vi "Read String IN.vi"(8 "error in (no error)":errorcluster, 11 "XuLyStringUART in":refnum<class "XuLyStringUART.lvclass">) -> (0 "error out":errorcluster, 2 "String IN":string, 3 "XuLyStringUART out":refnum<class "XuLyStringUART.lvclass">)   [LabVIEW 2017, in "LibraryGcode.lvlib" / "XuLyStringUART.lvclass"]
uses:
  XuLyStringUART.lvclass
  XuLyStringUART.lvclass/XuLyStringUART.ctl
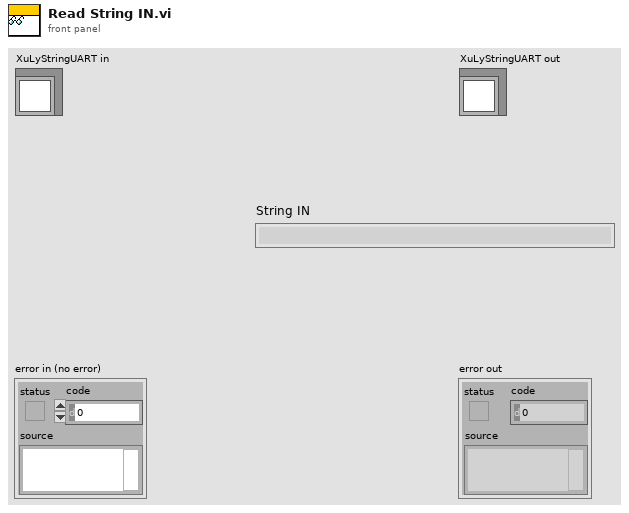
[diagram p1: front panel]
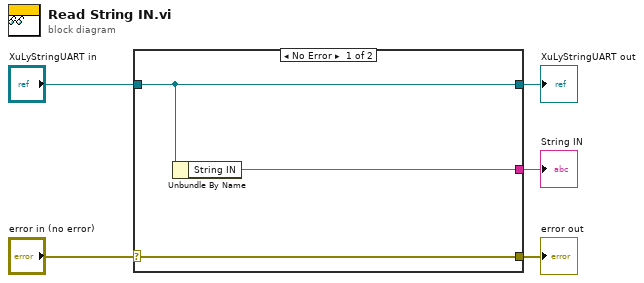
[diagram p0: block diagram]
diagram:
  n1 = case shown="No Error" "error in (no error)" {
    selector: "error in (no error)" -> [w8 w9]
    tunnel: [w8 w9] -> w4
    tunnel: [w7 w10] -> w2
    tunnel: "XuLyStringUART in" -> [w7 w10]
    tunnel: [w6 _] -> w1
    frame No Error {
      n2 = Unbundle By Name(w7) -> ("String IN"=w6:string)
    }
    frame Error {
    }
  }
  "error out" <- w4
  "XuLyStringUART out" <- w2
  "String IN" <- w1
